vi "Image acquisition color 16-bit RGB data - polling.vi"() -> ()   [LabVIEW 2015]
uses:
  C:/code/Host/Installer/Scientific Camera Interfaces/LabVIEW/64_bit/Library_X64/Thorlabs.TSI.TLCameraInterfaces.dll
  code/Host/Installer/Scientific Camera Interfaces/LabVIEW/64_bit/Library_X64/Thorlabs.TSI.TLCameraInterfaces.dll
  SubVIs/Parameters Get & Set/Set Parameters/Set Gain.vi
  SubVIs/Parameters Get & Set/Get Parameters/Get CameraSensorType.vi
  C:/code/Host/Installer/Scientific Camera Interfaces/LabVIEW/64_bit/Library_X64/Thorlabs.TSI.ColorInterfaces.dll
  code/Host/Installer/Scientific Camera Interfaces/LabVIEW/64_bit/Library_X64/Thorlabs.TSI.ColorInterfaces.dll
  C:/code/Host/Installer/Scientific Camera Interfaces/LabVIEW/64_bit/Library_X64/Thorlabs.TSI.ColorProcessor.dll
  code/Host/Installer/Scientific Camera Interfaces/LabVIEW/64_bit/Library_X64/Thorlabs.TSI.ColorProcessor.dll
  C:/code/Host/Installer/Scientific Camera Interfaces/LabVIEW/64_bit/Library_X64/Thorlabs.TSI.Demosaicker.dll
  code/Host/Installer/Scientific Camera Interfaces/LabVIEW/64_bit/Library_X64/Thorlabs.TSI.Demosaicker.dll
  SubVIs/Color/Color Processor References.ctl
  SubVIs/Parameters Get & Set/Get Parameters/Get BitDepth.vi
  SubVIs/Parameters Get & Set/Set Parameters/Set ExposureTime_us.vi
  SubVIs/Parameters Get & Set/Set Parameters/Set FramesPerTrigger_zeroForUnlimited.vi
  SubVIs/Parameters Get & Set/Set Parameters/Set OperationMode.vi
  SubVIs/Parameters Get & Set/Get Parameters/Get NumberOfQueuedFrames.vi
  C:/code/Host/Installer/Scientific Camera Interfaces/LabVIEW/64_bit/Library_X64/Thorlabs.TSI.ImageDataInterfaces.dll
  code/Host/Installer/Scientific Camera Interfaces/LabVIEW/64_bit/Library_X64/Thorlabs.TSI.ImageDataInterfaces.dll
  SubVIs/Parameters Get & Set/Get Parameters/Get ColorFilterArrayPhase.vi
  Controls/Color Balance.ctl
  Controls/Color Modes.ctl
panel:
  in  "Image Type":T1
  in  "Color Balance":T2={"Red Gain"=1.0, "Green Gain"=1.0, "Blue Gain"=1.0} {"Blue Gain" min=0 max=10 step=0.05 scale=0.0..10.0 scale format="%#_3g"; "Green Gain" min=0 max=10 step=0.05 scale=0.0..10.0 scale format="%#_3g"; "Red Gain" min=0 max=10 step=0.05 scale=0.0..10.0 scale format="%#_3g"}
  in  "Exposure (ms)":u32=100
  in  "Gain":u32 max=1023
  in  "Tab Control":T3(tab)
  out "Red Intensity Graph":u16[][](graph)
  out "Green Intensity Graph":u16[][](graph)
  out "Blue Intensity Graph":u16[][](graph)
  in  "stop":bool
  out "FrameNumber":u32
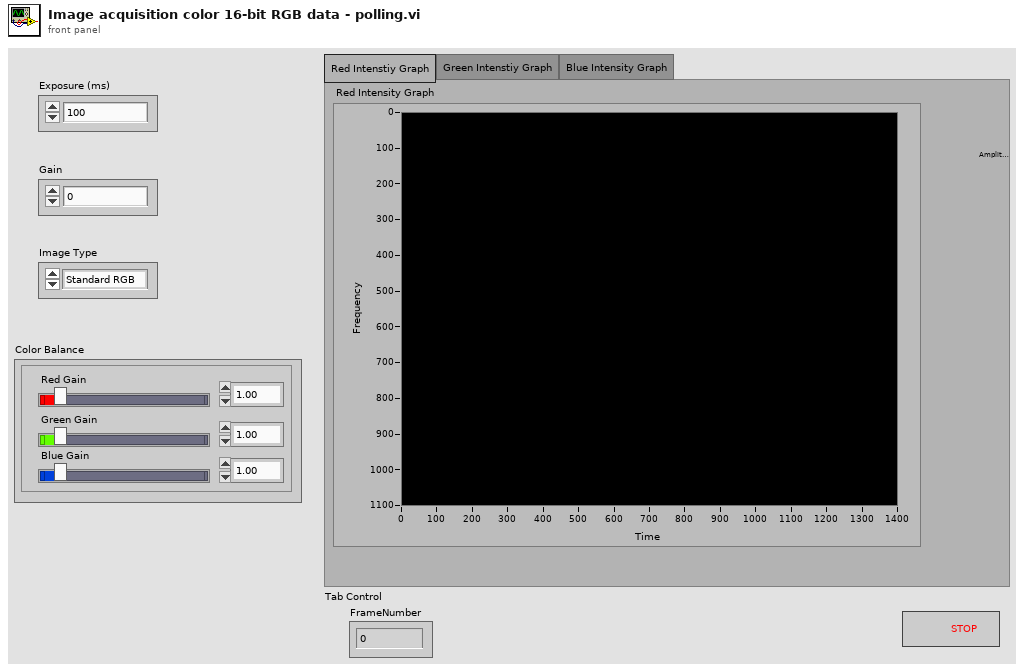
[diagram p1: front panel]
types:
  T1 = typedef "Color Modes.ctl" = enum16{"Standard RGB", "Linear RGB", "Unprocessed"}
  T2 = typedef "Color Balance.ctl" = cluster{"Red Gain":sgl, "Green Gain":sgl, "Blue Gain":sgl}
  T3 = enum32{"Red Intenstiy Graph", "Green Intenstiy Graph", "Blue Intensity Graph"}
  T4 = typedef "Color Processor References.ctl" = cluster{"Demosaicker reference":refnum<k24>, "ColorProcessorSDK reference":refnum<k24>, "StandardRGBColorProcessor":refnum<k24>, "LinearRGBColorProcessor":refnum<k24>}
  T5 = enum8{"Enabled", "Disabled", "Disabled and Grayed Out"}
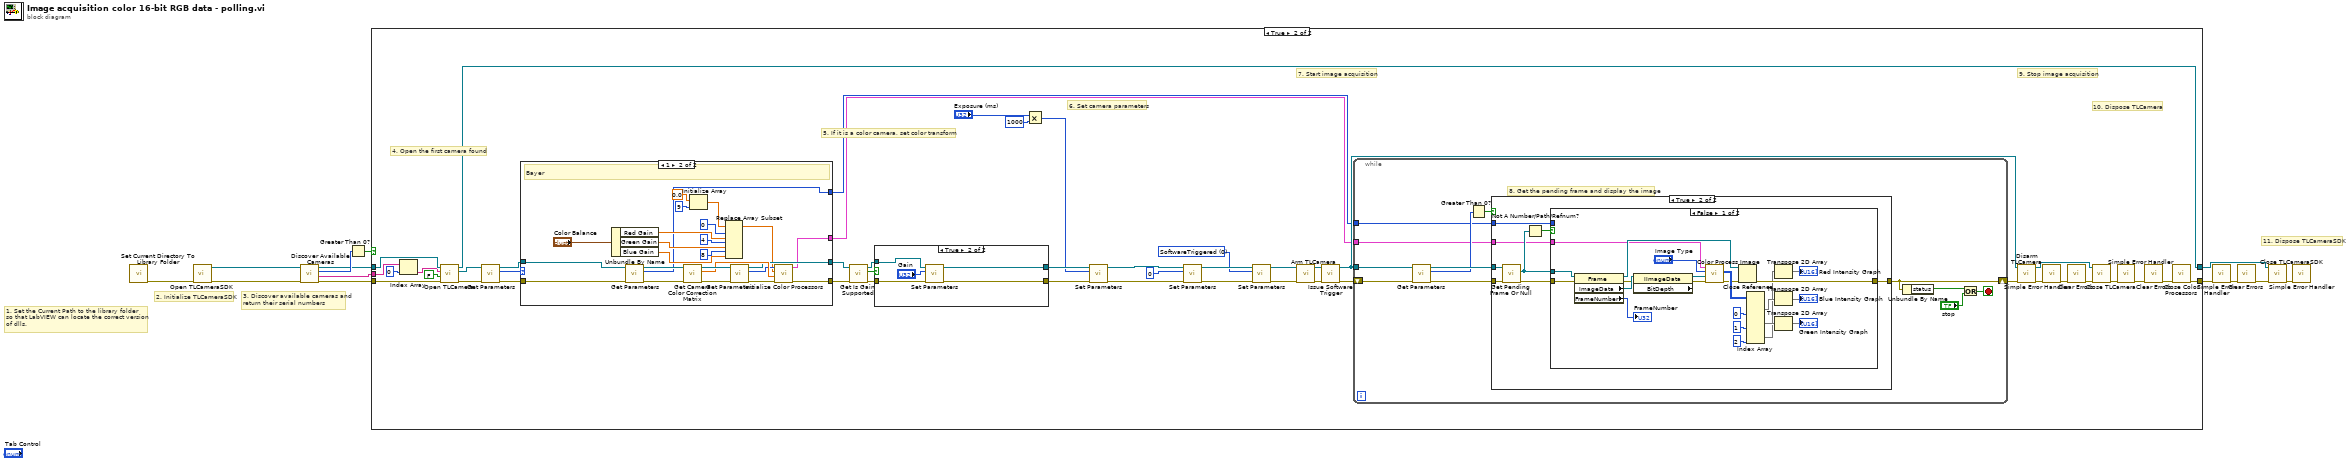
[diagram p0: block diagram]
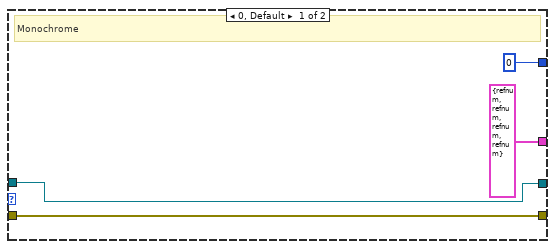
[diagram p3: hidden frame]
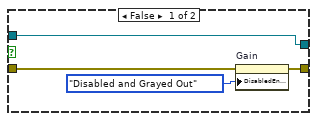
[diagram p4: hidden frame]
diagram:
  # "1. Set the Current Path to the library folder\nso that LabVIEW can locate the correct version\nof dlls."
  # "11. Dispose TLCameraSDK"
  # "3. Discover available cameras and\nreturn their serial numbers"
  # "2. Initialize TLCameraSDK"
  n1 = call "Set Current Directory To Library Folder.vi"() -> ("error out"=w8:errorcluster)  [unwired: 11 in]
  n2 = call "Open TLCameraSDK.vi"("error in (no error)"=w8) -> ("error out"=w7:errorcluster, "TLCameraSDK ref out"=w6:refnum<k24>)  [unwired: 9 in]
  n3 = call "Discover Available Cameras.vi"("error in (no error)"=w7, "TLCameraSDK reference"=w6) -> ("error out"=w12:errorcluster, "Serial Numbers"=w9:string[], "Number of Cameras"=w11:i32, "TLCameraSDK reference out"=w10:refnum<k24>)  [unwired: 6 in]
  n4 = Greater Than 0?(x=w11) -> (x > 0?=w13:bool)
  n5 = case shown="True" w13 {
    tunnel: w10 -> [w14 w60]
    tunnel: w12 -> [w15 w46]
    tunnel: [w15 w21] -> w1
    tunnel: [w14 w58] -> w2
    tunnel: w9 -> [_ w56]
    frame False {
    }
    frame True {
      w32 = 0 items=["SoftwareTriggered", "HardwareTriggered", "Bulb", "Reserved1", "Reserved2"] ("OperationMode")
      # "10. Dispose TLCamera"
      # "9. Stop image acquisition"
      # "7. Start image acquisition"
      # "6. Set camera parameters"
      # "5. If it is a color camera, set color transform"
      # "4. Open the first camera found"
      n6 = Index Array(array=w56, index=0) -> (element=w47:string)
      n7 = call "Open TLCamera.vi"("error in (no error)"=w46, "isDiagnosticsMessagesEnabled"=FALSE, "Camera serial number"=w47, "TLCameraSDK reference"=w60) -> ("error out"=w44:errorcluster, "TLCamera reference out"=w45:refnum<k24>, "TLCameraSDK reference out"=w58:refnum<k24>)  [unwired: 5 in]
      n8 = call-poly "Get Parameters.vi"("error in (no error)"=w44, "TLCamera reference in"=w45) -> ("error out"=w42:errorcluster, "CameraSensorType"=w43:i32, "TLCamera reference out"=w41:refnum<k24>)  [unwired: 7 in]
      n9 = case shown="1" w43 {
        tunnel: w41 -> [w63 w69]
        tunnel: w42 -> [w64 w67]
        tunnel: [w64 w73] -> w40
        tunnel: [w63 w74] -> w39
        tunnel: [T4 {"Demosaicker reference"=refnum, "ColorProcessorSDK reference"=refnum, "StandardRGBColorProcessor"=refnum, "LinearRGBColorProcessor"=refnum} ("Color Processor References") w72] -> w19
        tunnel: [0 ("ColorFilterArrayPhase") w65] -> w18
        frame 0, Default {
          # "Monochrome"
        }
        frame 1 {
          # "Bayer"
          n10 = Unbundle By Name("Color Balance") -> ("Red Gain"=w84:sgl, "Green Gain"=w86:sgl, "Blue Gain"=w88:sgl)
          n11 = call-poly "Get Parameters.vi"("error in (no error)"=w67, "TLCamera reference in"=w69) -> ("error out"=w66:errorcluster, "ColorFilterArrayPhase"=w65:i32, "TLCamera reference out"=w68:refnum<k24>)  [unwired: 7 in]
          n12 = call "Get Camera Color Correction Matrix.vi"("error in (no error)"=w66, "TLCamera reference"=w68) -> ("error out"=w78:errorcluster, "Camera Color Correction Matrix"=w75:sgl[], "TLCamera reference out"=w77:refnum<k24>)  [unwired: 7 in]
          n13 = Initialize Array(sgl 0.0 ("element"), 9 ("dimension size")) -> (w81:sgl[])
          n14 = Replace Array Subset(array=w81, new element #1=w84, index #1=0 ("index"), new element #2=w86, index #2=4 ("index"), new element #3=w88, index #3=8 ("index")) -> (w70:sgl[])
          n15 = call-poly "Get Parameters.vi"("error in (no error)"=w78, "TLCamera reference in"=w77) -> ("error out"=w76:errorcluster, "BitDepth"=w71:u32, "TLCamera reference out"=w74:refnum<k24>)  [unwired: 7 in]
          n16 = call "Initialize Color Processors.vi"("error in (no error)"=w76, "Camera Color Correction Matrix"=w75, "White Balance Matrix"=w70, "BitDepth"=w71) -> ("error out"=w73:errorcluster, "Color Processor References"=w72:T4)  [unwired: 6 in]
        }
      }
      n17 = call "Get Is Gain Supported.vi"("error in (no error)"=w40, "TLCamera reference in"=w39) -> ("error out"=w51:errorcluster, "Is Gain Supported?"=w53:bool, "TLCamera reference out"=w52:refnum<k24>)  [unwired: 7 in]
      n18 = case shown="True" w53 {
        tunnel: w52 -> [w89 w95]
        tunnel: w51 -> [w90 w97]
        tunnel: [w91 w96] -> w37
        tunnel: [w89 w94] -> w50
        frame False {
          n19 = property on="Gain" class="DigNum (strict)"(error in=w90, "DisabledEnum"=T5."Disabled and Grayed Out" ("Disabled")) -> (error out=w91:errorcluster)  [unwired: 1 in, 1 out]
        }
        frame True {
          n20 = call-poly "Set Parameters.vi"("error in (no error)"=w97, "Gain"="Gain", "TLCamera reference in"=w95) -> ("error out"=w96:errorcluster, "TLCamera reference out"=w94:refnum<k24>)  [unwired: 7 in]
        }
      }
      n21 = Multiply(x="Exposure (ms)", y=u32 1000) -> (x*y=w31:u32)
      n22 = call-poly "Set Parameters.vi"("error in (no error)"=w37, "ExposureTime_us"=w31, "TLCamera reference in"=w50) -> ("error out"=w35:errorcluster, "TLCamera reference out"=w36:refnum<k24>)  [unwired: 7 in]
      n23 = call-poly "Set Parameters.vi"("error in (no error)"=w35, "FramesPerTrigger_zeroForUnlimited"=u32 0 ("FramesPerTriggerOrZeroForUnlimited"), "TLCamera reference in"=w36) -> ("error out"=w33:errorcluster, "TLCamera reference out"=w34:refnum<k24>)  [unwired: 7 in]
      n24 = call-poly "Set Parameters.vi"("error in (no error)"=w33, "OperationMode"=w32, "TLCamera reference in"=w34) -> ("error out"=w16:errorcluster, "TLCamera reference out"=w17:refnum<k24>)  [unwired: 7 in]
      n25 = call "Arm TLCamera.vi"("error in (no error)"=w16, "TLCamera reference"=w17) -> ("error out"=w30:errorcluster, "TLCamera reference out"=w54:refnum<k24>)  [unwired: 8 in]
      n26 = call "Issue Software Trigger.vi"("error in (no error)"=w30, "TLCamera Reference"=w54) -> ("error out"=w55:errorcluster, "TLCamera reference out"=w20:refnum<k24>)  [unwired: 8 in]
      n27 = while {
        tunnel: w20 -> [w109]
        shift-right: [w106] -> w22
        shift-left: w55 -> [w102]
        tunnel: w18 -> [w99]
        tunnel: w19 -> [w98]
        stop <- w103 stop-if-true
        # "8. Get the pending frame and display the image"
        n28 = call-poly "Get Parameters.vi"("error in (no error)"=w102, "TLCamera reference in"=w109) -> ("error out"=w101:errorcluster, "NumberOfQueuedFrames"=w100:i32, "TLCamera reference out"=w107:refnum<k24>)  [unwired: 7 in]
        n29 = Greater Than 0?(x=w100) -> (x > 0?=w108:bool)
        n30 = case shown="True" w108 {
          tunnel: w101 -> [w110 w115]
          tunnel: w107 -> [_ w118]
          tunnel: [w110 w116] -> w106
          tunnel: w99 -> [_ w112]
          tunnel: w98 -> [_ w111]
          frame False {
          }
          frame True {
            n31 = call "Get Pending Frame Or Null.vi"("error in (no error)"=w115, "TLCamera reference"=w118) -> ("error out"=w114:errorcluster, "Pending Frame Or Null"=w113:refnum<k24>)  [unwired: 7 in, 1 out]
            n32 = Not A Number/Path/Refnum?(number/path/refnum=w113) -> (NaN/Path/Refnum?=w117:bool)
            n33 = case shown="False" w117 {
              tunnel: w113 -> [w140 _]
              tunnel: w114 -> [w139 w141]
              tunnel: [w137 w141] -> w116
              tunnel: w112 -> [_ _]
              tunnel: w111 -> [w121 _]
              frame False {
                n34 = property class="Frame"(reference=w140, error in=w139) -> (reference out=w138:refnum<k24>, error out=w134:errorcluster, "ImageData"=w135:refnum<k24>, "FrameNumber"=→"FrameNumber":u32)
                n35 = property class="IImageData" props=["BitDepth"](reference=w135, error in=w134) -> (reference out=w124:refnum<k24>, error out=w122:errorcluster)  [unwired: 1 out]
                n36 = call "Color Process Image.vi"("error in (no error)"=w122, "ImageData"=w124, "Image Type"="Image Type", "Color Processor References"=w121) -> ("error out"=w119:errorcluster, "Color Data"=w120:u16[][][])  [unwired: 6 in]
                n37 = Close Reference(reference=w138, error in (no error)=w119) -> (error out=w137:errorcluster)
                n38 = Index Array(array=w120, index (dim 2) #1=0 ("disabled index (col)"), index (dim 2) #2=1 ("index (col)"), index (dim 2) #3=2 ("index (col)")) -> (element #1=w130:u16[][], element #2=w128:u16[][], element #3=w126:u16[][])  [unwired: 6 in]
                n39 = Transpose 2D Array(2D array=w126) -> (transposed array=→"Red Intensity Graph":u16[][])
                n40 = Transpose 2D Array(2D array=w130) -> (transposed array=→"Blue Intensity Graph":u16[][])
                n41 = Transpose 2D Array(2D array=w128) -> (transposed array=→"Green Intensity Graph":u16[][])
              }
              frame True {
              }
            }
          }
        }
        n42 = Unbundle By Name(w106) -> ("status"=w104:bool)
        n43 = Or(x=w104, y="stop") -> (x .or. y?=w103:bool)
      }
      n44 = call "Disarm TLCamera.vi"("error in (no error)"=w22, "TLCamera reference"=w20) -> ("error out"=w28:errorcluster, "TLCamera reference out"=w29:refnum<k24>)  [unwired: 8 in]
      n45 = call <vilib>:"Simple Error Handler.vi"("error in (no error)"=w28) -> ("error out"=w27:errorcluster)  [unwired: 4 in, 4 out]
      n46 = call <vilib>:"Clear Errors.vi"("error in (no error)"=w27) -> ("error out"=w26:errorcluster)  [unwired: 5 in, 1 out]
      n47 = call "Close TLCamera.vi"("error in (no error)"=w26, "TLCamera reference"=w29) -> ("error out"=w24:errorcluster)  [unwired: 9 in]
      n48 = call <vilib>:"Simple Error Handler.vi"("error in (no error)"=w24) -> ("error out"=w25:errorcluster)  [unwired: 4 in, 4 out]
      n49 = call <vilib>:"Clear Errors.vi"("error in (no error)"=w25) -> ("error out"=w23:errorcluster)  [unwired: 5 in, 1 out]
      n50 = call "Close Color Processors.vi"("error in (no error)"=w23) -> ("error out"=w21:errorcluster)  [unwired: 10 in]
    }
  }
  n51 = call <vilib>:"Simple Error Handler.vi"("error in (no error)"=w1) -> ("error out"=w4:errorcluster)  [unwired: 4 in, 4 out]
  n52 = call <vilib>:"Clear Errors.vi"("error in (no error)"=w4) -> ("error out"=w3:errorcluster)  [unwired: 5 in, 1 out]
  n53 = call "Close TLCameraSDK.vi"("error in (no error)"=w3, "TLCameraSDK reference"=w2) -> ("error out"=w5:errorcluster)  [unwired: 9 in]
  n54 = call <vilib>:"Simple Error Handler.vi"("error in (no error)"=w5) -> ()  [unwired: 4 in, 5 out]
